vi "FTW-Actor-Broker-Destroy.vi"(0 "FTW Message Broker":refnum<class "FTW-Actor-Broker.lvclass">, 11 "error in":errorcluster) -> (15 "error out":errorcluster)   [LabVIEW 2013, in "FTW-Actor-Broker.lvclass"]
uses:
  FTW-Actor-Broker.lvclass
panel:
  # "Inputs"
  # "Outputs"
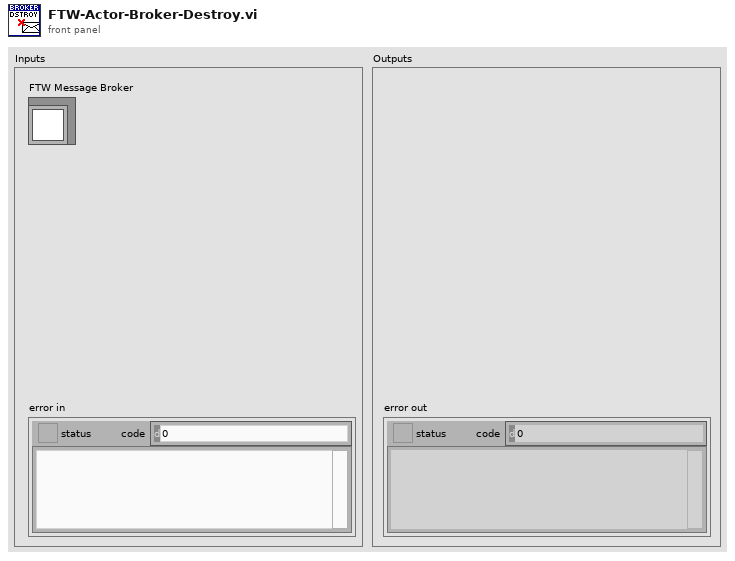
[diagram p1: front panel]
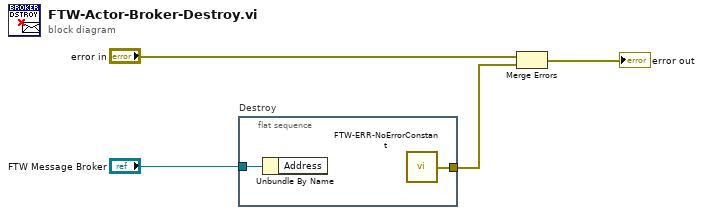
[diagram p0: block diagram]
diagram:
  n1 = flat-sequence "Destroy" {
    tunnel: "FTW Message Broker" -> [w6]
    tunnel: [w5] -> w1
    frame #0 {
      n2 = Unbundle By Name(w6) -> ()  [unwired: 1 out]
      n3 = call "FTW-ERR-NoErrorConstant.vi"() -> ("no error"=w5:errorcluster)
    }
  }
  n4 = Merge Errors("error in", w1) -> (→"error out":errorcluster)
